vi "ObtainSettingsQueue.vi"(8 "error in (no error)":errorcluster) -> (0 "error out":errorcluster, 3 "Queue out":refnum<queue>)   [LabVIEW 2019, in "Settings.lvlib"]
uses:
  Settings.lvlib
  CTL_MessageCluster.ctl
  CTL_SettingsMessage.ctl
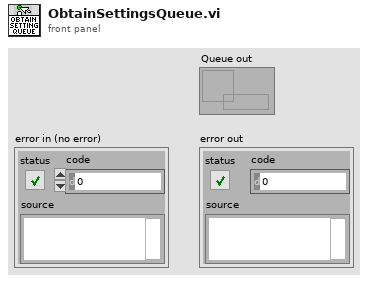
[diagram p1: front panel]
types:
  T1 = typedef "Settings.lvlib/CTL_MessageCluster.ctl" = cluster{"Message":T2, "Data":variant}
  T2 = typedef "Settings.lvlib/CTL_SettingsMessage.ctl" = enum16{"Inititalize", "Idle", "LoadSettings", "SaveSettings", "Exit"}
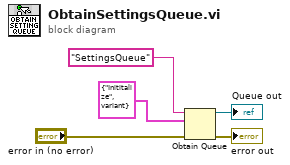
[diagram p0: block diagram]
diagram:
  n1 = Obtain Queue(name (unnamed)="SettingsQueue", element data type=T1 {"Message"=enum."Inititalize", "Data"=variant} ("SettingsMessage"), error in (no error)="error in (no error)") -> (queue out=→"Queue out":refnum<queue>, error out=→"error out":errorcluster)  [unwired: 2 in, 1 out]
